vi "convert RegisterMap to FPGA Scalar.vi"(8 "error in":errorcluster, 11 "RegisterMap":T1[](array[typedef]) {"Address" format="%.0x"}) -> (0 "error out":errorcluster, 3 "FPGA Scalar":T6[](array[typedef]) {"Data Type" format="%.0x"})   [LabVIEW 2016, in "FPGA Addon Shared.lvlib"]
uses:
  Shared/FPGA Addon Shared.lvlib
  Shared/Register Information.ctl
  Shared/Data Type.ctl
  <vilib>/rvi/Bitfile/nirviControlStructure.ctl
  <vilib>/rvi/Bitfile/nirviTypdefDescription.ctl
  <vilib>/rvi/Bitfile/nirviMechanicalAction.ctl
  <vilib>/rvi/Bitfile/nirviSubControlStructure.ctl
  <vilib>/rvi/Bitfile/nirviClusterElementControl.ctl
  FPGA/Speciality IO/Types/PWM.Measure.Analog.Measurement.ctl
  FPGA/Speciality IO/Types/PWM.Measure.Digital.Measurement.ctl
  FPGA/Speciality IO/Types/PWM.Generate.Digital.Settings.ctl
  FPGA/Speciality IO/Types/PWM.Measure.Analog.Settings.ctl
  FPGA/Speciality IO/Types/PWM.Measure.Digital.Settings.ctl
  FPGA/Speciality IO/Types/Sine.Generate.Settings.ctl
  FPGA/Speciality IO/Speciality FPGA IO.lvlib
  <vilib>/Utility/Data Type/NI_Data Type.lvlib
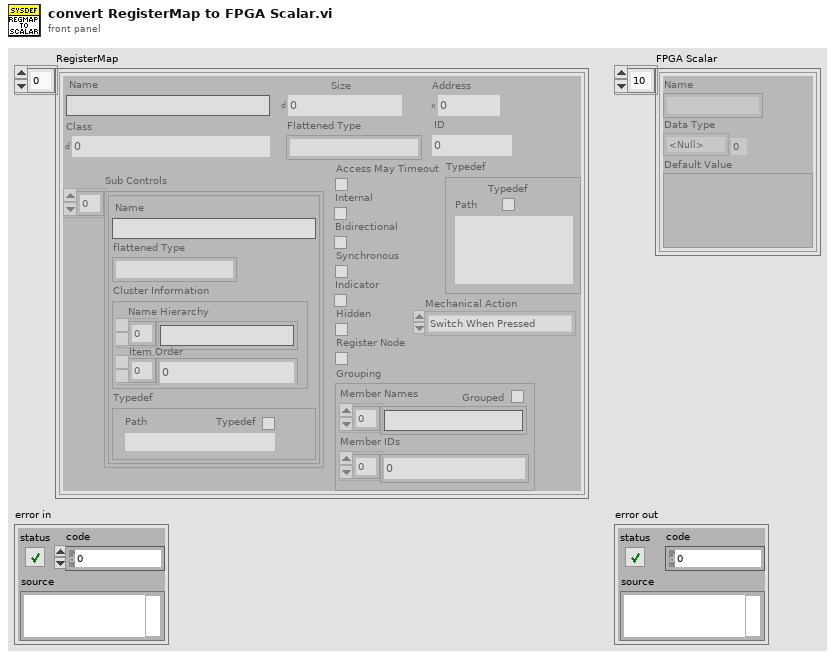
[diagram p1: front panel]
types:
  T1 = typedef "nirviControlStructure.ctl" = cluster{"Name":string, "Hidden":bool, "Indicator":bool, "Flattened Type":string, "Grouping":cluster{"Grouped":bool, "Member Names":string[], "Member IDs":u32[]}, "Address":u32, "Size":u32, "Class":u32, "Internal":bool, "Typedef":T2, "ID":u32, "Bidirectional":bool, "Synchronous":bool, "Mechanical Action":T3, "Sub Controls":T4[], "Access May Timeout":bool, "Register Node":bool}
  T2 = typedef "nirviTypdefDescription.ctl" = cluster{"Typedef":bool, "Path":path}
  T3 = typedef "nirviMechanicalAction.ctl" = enum8{"Switch When Pressed", "Switch When Released", "Switch Until Released", "Latch When Pressed", "Latch When Released", "Latch Until Released"}
  T4 = typedef "nirviSubControlStructure.ctl" = cluster{"Name":string, "flattened Type":string, "Cluster Information":T5, "Typedef":T2}
  T5 = typedef "nirviClusterElementControl.ctl" = cluster{"Name Hierarchy":string[], "Item Order":u32[]}
  T6 = typedef "FPGA Addon Shared.lvlib/Register Information.ctl" = cluster{"Name":string, "Data Type":T7, "Default Value":variant}
  T7 = typedef "FPGA Addon Shared.lvlib/Data Type.ctl" = enum8{"<Null>", "I8", "I16", "I32", "I64", "U8", "U16", "U32", "U64", "SGL", "Boolean", "Analog PWM In Settings", "Analog PWM In", "Digital PWM In Settings", "Digital PWM In", "Digital PWM Out", "Sine Out", "FXP+/-24.5", "FXP+/-16.5", "FXP+/-32.8", "FXP+/-64.32", "FXP+/-16.7", "FXP+/-20.5"}
  T8 = typedef "Speciality FPGA IO.lvlib/PWM.Measure.Digital.Measurement.ctl" = cluster{"ACTIVE TICKS":u32, "INACTIVE TICKS":u32, "ACQ TICKS":u32}
  T9 = typedef "Speciality FPGA IO.lvlib/PWM.Measure.Analog.Measurement.ctl" = cluster{"ACTIVE TICKS":u32, "INACTIVE TICKS":u32, "ACQ TICKS":u32, "ACTIVE VOLTAGE":fxp<+/-,32,8>, "INACTIVE VOLTAGE":fxp<+/-,32,8>}
  T10 = typedef "Speciality FPGA IO.lvlib/Sine.Generate.Settings.ctl" = cluster{"AMP":fxp<+/-,32,8>, "OFFSET":fxp<+/-,32,8>, "PERIODS/TICKS":fxp<+,32,0>}
  T11 = typedef "Speciality FPGA IO.lvlib/PWM.Measure.Digital.Settings.ctl" = cluster{"ACTIVE EDGE":bool, "TIMEOUT":u32}
  T12 = typedef "Speciality FPGA IO.lvlib/PWM.Measure.Analog.Settings.ctl" = cluster{"ACTIVE EDGE":bool, "TIMEOUT":u32, "THRESHOLD":fxp<+/-,32,8>}
  T13 = typedef "Speciality FPGA IO.lvlib/PWM.Generate.Digital.Settings.ctl" = cluster{"ACTIVE EDGE":bool, "ACTIVE TICKS":u32, "INACTIVE TICKS":u32}
  T14 = typedef "NI_Data Type.lvlib/Data Type.ctl" = enum8{"Invalid Type", "Void", "I8", "I16", "I32", "I64", "U8", "U16", "U32", "U64", "Single Float", "Double Float", "Extended Float", "Single Complex", "Double Complex", "Extended Complex", "Enum U8", "Enum U16", "Enum U32", "Enum U64", "Single Float With Unit", "Double Float With Unit", "Extended Float With Unit", "Single Complex with Unit", "Double Complex with Unit", "Extended Complex with Unit", "Boolean", "String", "Path", "Picture", "Tag", "Array", "Cluster", "Variant", "LV Variant", "Waveform", "Timestamp", "Digital Waveform", "Digital Data", "ExpressData", "Refnum", "External Data", "VI", "Poly VI", "LabVIEW Class Instance", "Fixed Point"}
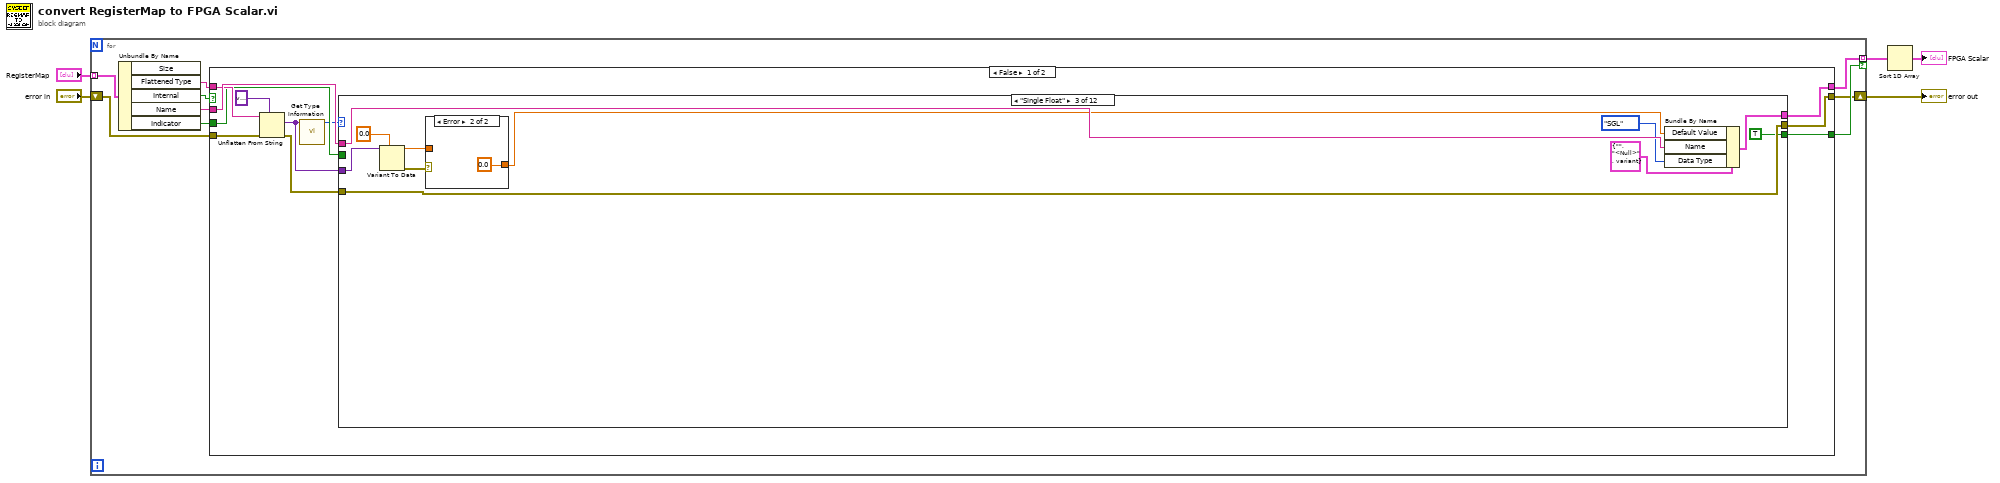
[diagram p0: block diagram]
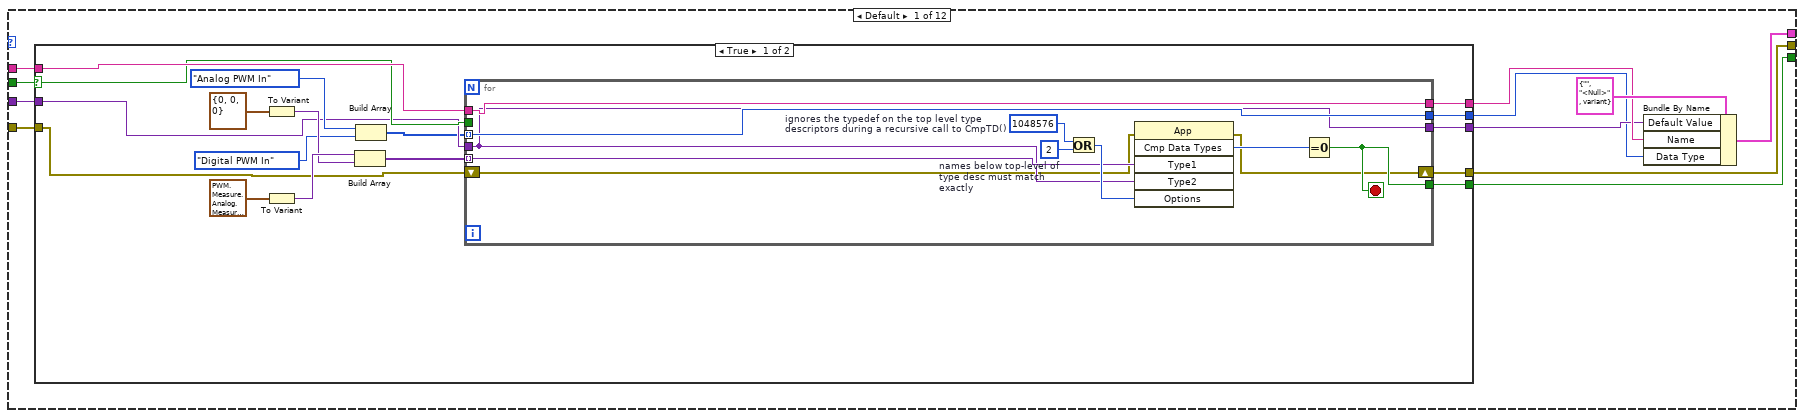
[diagram p2: hidden frame]
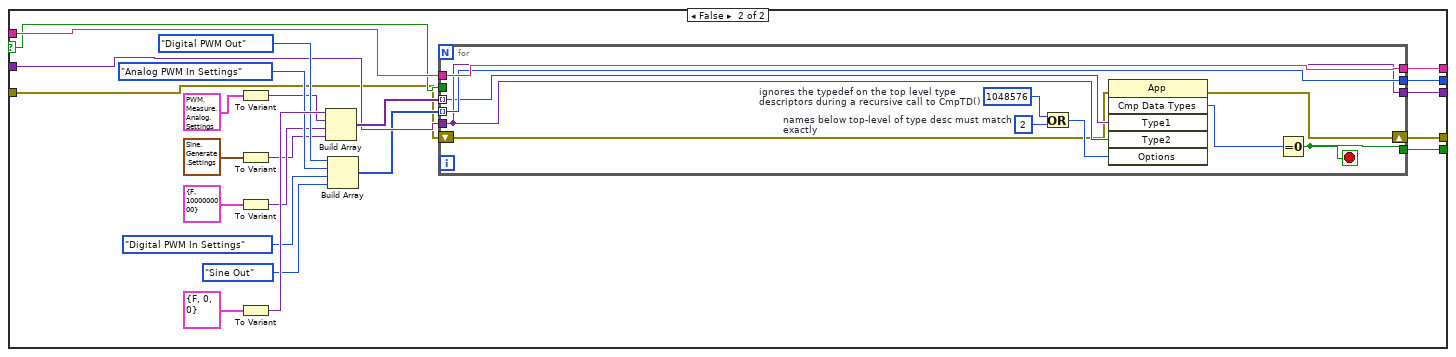
[diagram p3: hidden frame]
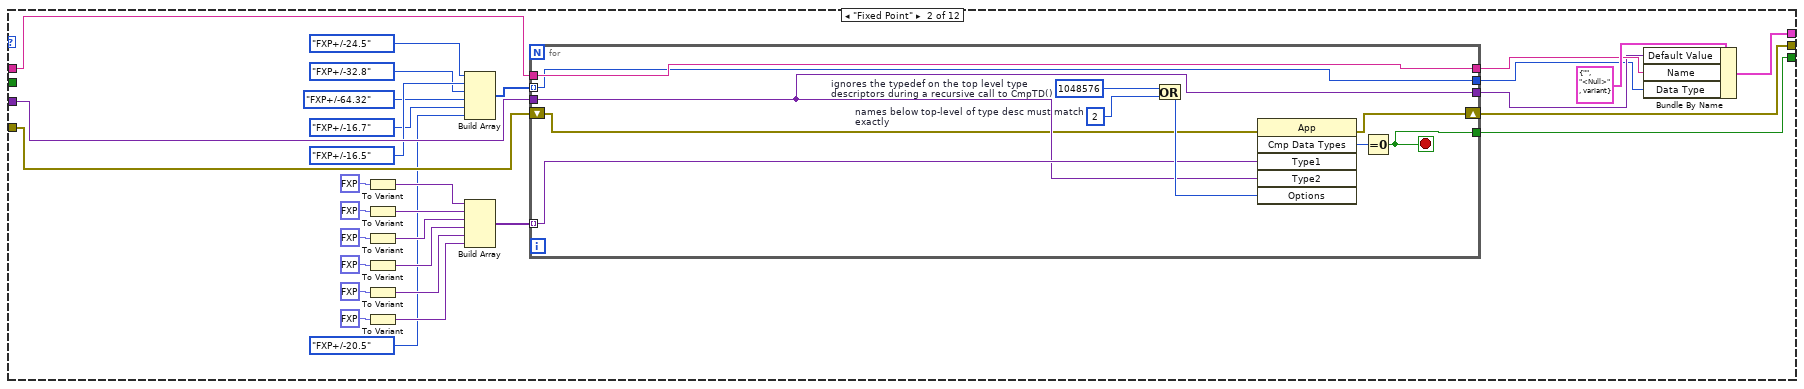
[diagram p4: hidden frame]
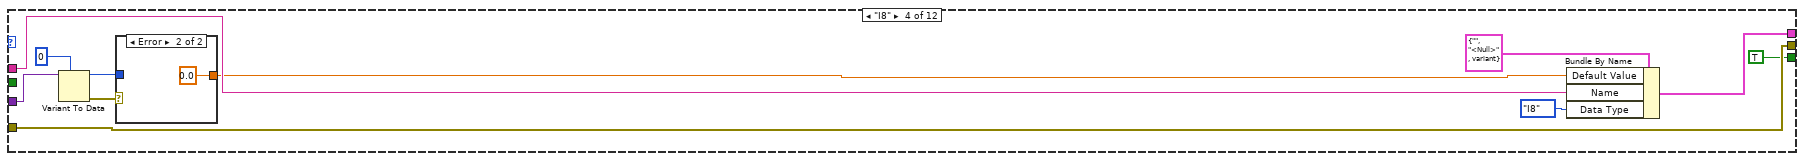
[diagram p6: hidden frame]
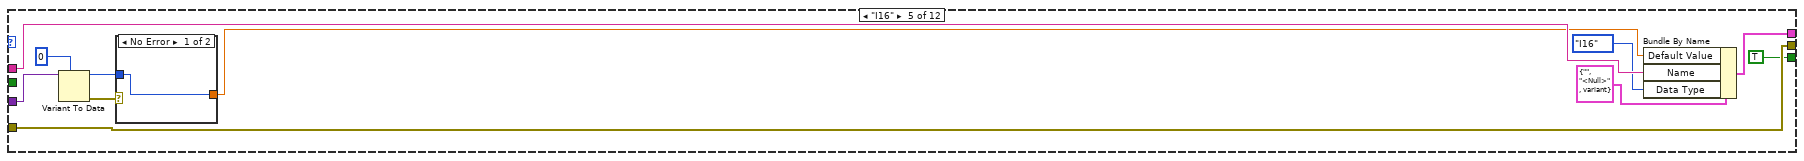
[diagram p8: hidden frame]
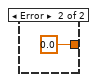
[diagram p9: hidden frame]
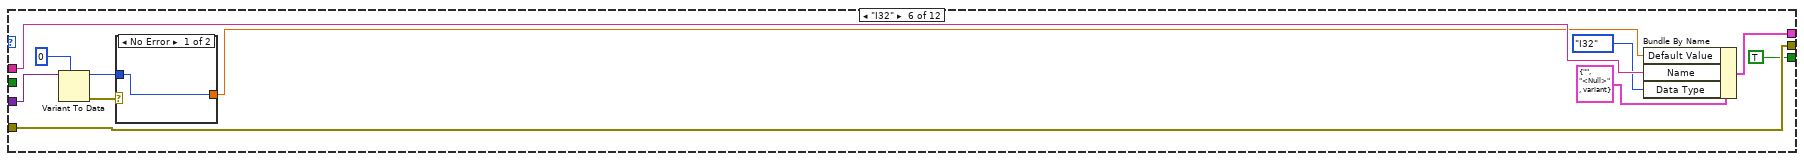
[diagram p10: hidden frame]
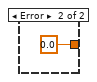
[diagram p11: hidden frame]
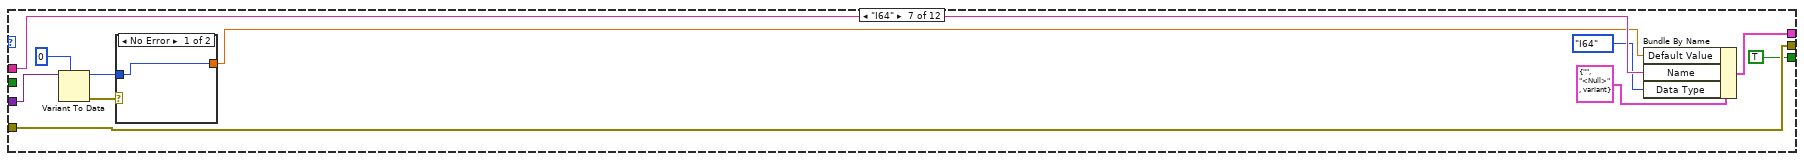
[diagram p12: hidden frame]
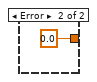
[diagram p13: hidden frame]
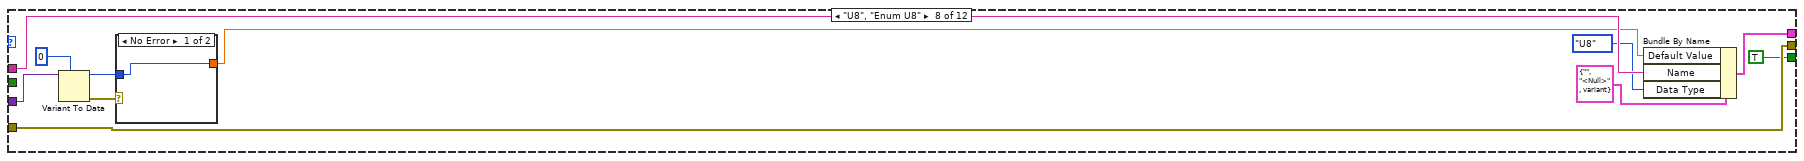
[diagram p14: hidden frame]
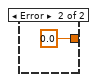
[diagram p15: hidden frame]
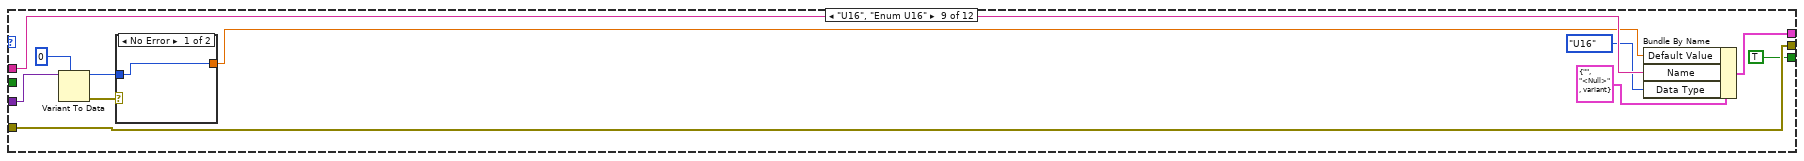
[diagram p16: hidden frame]
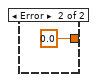
[diagram p17: hidden frame]
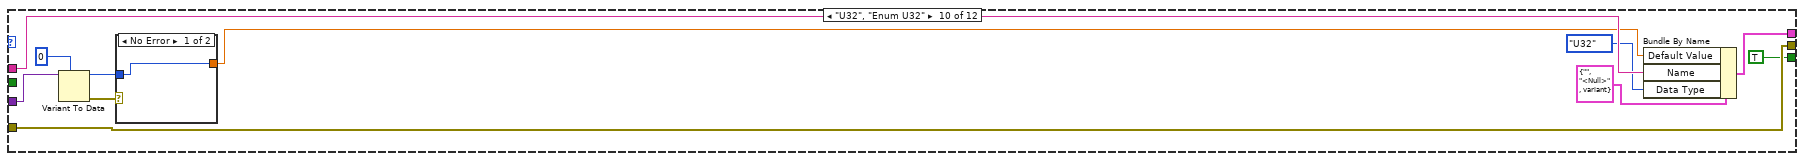
[diagram p18: hidden frame]
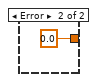
[diagram p19: hidden frame]
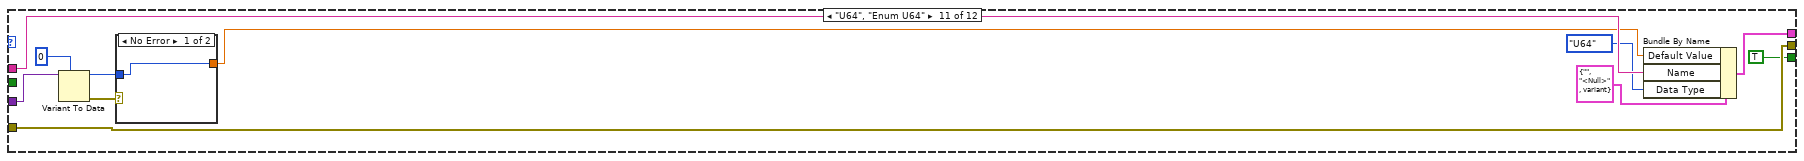
[diagram p20: hidden frame]
diagram:
  n1 = for {
    tunnel: "RegisterMap" -> [w10] mode=indexing
    tunnel: [w14] -> w5 mode=indexing if=w13
    shift-right: [w12] -> w3
    shift-left: "error in" -> [w11]
    n2 = Unbundle By Name(w10) -> ("Flattened Type"=w7:string, "Internal"=w8:bool, "Name"=w9:string, "Indicator"=w6:bool)  [unwired: 1 out]
    n3 = case shown="False" w8 {
      tunnel: w9 -> [w25 _]
      tunnel: [w24 _] -> w14
      tunnel: [w23 FALSE ("Boolean")] -> w13
      tunnel: w7 -> [w20 _]
      tunnel: [w22 w271] -> w12
      tunnel: w11 -> [w19 w271]
      tunnel: w6 -> [w17 _]
      frame False {
        n4 = Unflatten From String(type=variant ("Variant"), binary string=w20, error in (no error)=w19) -> (value=w16:variant, error out=w18:errorcluster)  [unwired: 3 out]
        n5 = call <vilib>:"Get Type Information.vi"("Variant"=w16) -> ("Type"=w15:T14)  [unwired: 6 in, 4 out]
        n6 = case shown="\"Single Float\"" w15 {
          tunnel: [w36 w128 TRUE ("Boolean") TRUE ("Boolean") TRUE ("Boolean") TRUE ("Boolean") TRUE ("Boolean") TRUE ("Boolean") TRUE ("Boolean") TRUE ("Boolean") TRUE ("Boolean") TRUE ("Boolean")] -> w23
          tunnel: w25 -> [w33 w125 w149 w162 w175 w188 w201 w214 w227 w240 w253 w266]
          tunnel: [w34 w126 w148 w161 w174 w187 w200 w213 w226 w239 w252 w265] -> w24
          tunnel: w16 -> [w32 w124 w147 w160 w173 w186 w199 w212 w225 w238 w251 w264]
          tunnel: [w28 w120 w141 w154 w167 w180 w193 w206 w219 w232 w245 w258] -> w22
          tunnel: w18 -> [w27 w119 w141 w154 w167 w180 w193 w206 w219 w232 w245 w258]
          tunnel: w17 -> [w26 _ _ _ _ _ _ _ _ _ _ _]
          frame Default {
            n7 = case shown="True" w26 {
              selector: w26 -> [w49 w84]
              tunnel: [w53 w87] -> w36
              tunnel: w33 -> [w52 w86]
              tunnel: w32 -> [w43 w80]
              tunnel: [w42 w79] -> w31
              tunnel: [w41 w78] -> w30
              tunnel: [w40 w77] -> w29
              tunnel: [w38 w68] -> w28
              tunnel: w27 -> [w37 w69]
              frame True {
                n8 = To Variant(anything=T8 {"ACTIVE TICKS"=0, "INACTIVE TICKS"=0, "ACQ TICKS"=0} ("Cached.Data")) -> (Variant=w47:variant)
                n9 = To Variant(anything=T9 {"ACTIVE TICKS"=0, "INACTIVE TICKS"=0, "ACQ TICKS"=0, "ACTIVE VOLTAGE"=0.0, "INACTIVE VOLTAGE"=0.0} ("Cached.Data")) -> (Variant=w48:variant)
                n10 = Build Array(w48, w47) -> (w44:variant[])
                n11 = Build Array(Data_Type."Analog PWM In" ("Data Type"), Data_Type."Digital PWM In" ("Data Type")) -> (w39:T7[])
                n12 = for {
                  tunnel: w43 -> [w57]
                  tunnel: w52 -> [w64]
                  tunnel: w44 -> [w59] mode=indexing
                  tunnel: [w57] -> w41
                  tunnel: [w64] -> w42
                  tunnel: [w63] -> w40
                  tunnel: w39 -> [w63] mode=indexing
                  tunnel: w49 -> [_]
                  tunnel: [w58] -> w53
                  shift-right: [w54] -> w38
                  shift-left: w37 -> [w55]
                  stop <- w58 stop-if-true
                  w56 = 2  # names below top-level of type desc must match exactly
                  w61 = 1048576  # ignores the typedef on the top level type descriptors during a recursive call to CmpTD()
                  n13 = Or(x=w61, y=w56) -> (x .or. y?=w62:i32)
                  n14 = invoke class="App" method="Cmp Data Types"(error in=w55, "Type1"=w59, "Type2"=w57, "Options"=w62) -> (error out=w54:errorcluster, "Compare Data Types"=w60:i32)  [unwired: 2 in, 4 out]
                  n15 = Equal To 0?(x=w60) -> (x = 0?=w58:bool)
                }
              }
              frame False {
                n16 = To Variant(anything=T12 {"ACTIVE EDGE"=FALSE, "TIMEOUT"=1000000000, "THRESHOLD"=3.0} ("Channel.Settings")) -> (Variant=w73:variant)
                n17 = To Variant(anything=T10 {"AMP"=0.0, "OFFSET"=0.0, "PERIODS/TICKS"=0.0002500000409781933} ("Settings")) -> (Variant=w66:variant)
                n18 = To Variant(anything=T11 {"ACTIVE EDGE"=FALSE, "TIMEOUT"=1000000000} ("Channel.Settings")) -> (Variant=w72:variant)
                n19 = To Variant(anything=T13 {"ACTIVE EDGE"=FALSE, "ACTIVE TICKS"=0, "INACTIVE TICKS"=0} ("Channel.Settings")) -> (Variant=w83:variant)
                n20 = Build Array(w83, w73, w72, w66) -> (w81:variant[])
                n21 = Build Array(Data_Type."Digital PWM Out" ("Data Type"), Data_Type."Analog PWM In Settings" ("Data Type"), Data_Type."Digital PWM In Settings" ("Data Type"), Data_Type."Sine Out" ("Data Type")) -> (w76:T7[])
                n22 = for {
                  tunnel: w80 -> [w93]
                  tunnel: w86 -> [w98]
                  tunnel: w81 -> [w92] mode=indexing
                  tunnel: [w93] -> w78
                  tunnel: [w98] -> w79
                  tunnel: [w97] -> w77
                  tunnel: w76 -> [w97] mode=indexing
                  tunnel: w84 -> [_]
                  tunnel: [w90] -> w87
                  shift-right: [w88] -> w68
                  shift-left: w69 -> [w89]
                  stop <- w90 stop-if-true
                  w95 = 2  # names below top-level of type desc must match exactly
                  w94 = 1048576  # ignores the typedef on the top level type descriptors during a recursive call to CmpTD()
                  n23 = Or(x=w94, y=w95) -> (x .or. y?=w96:i32)
                  n24 = invoke class="App" method="Cmp Data Types"(error in=w89, "Type1"=w92, "Type2"=w93, "Options"=w96) -> (error out=w88:errorcluster, "Compare Data Types"=w91:i32)  [unwired: 2 in, 4 out]
                  n25 = Equal To 0?(x=w91) -> (x = 0?=w90:bool)
                }
              }
            }
            n26 = Bundle By Name(cluster=T6 {"Name"="", "Data Type"=enum."<Null>", "Default Value"=variant(refnum<class> refnum)}, "Default Value"=w30, "Name"=w31, "Data Type"=w29) -> (w34:T6)
          }
          frame "Fixed Point" {
            n27 = To Variant(anything=fxp<+/-,24,5> 0.0 ("Numeric 1 In")) -> (Variant=w118:variant)
            n28 = To Variant(anything=fxp<+/-,16,5> 0.0 ("Numeric 2 In")) -> (Variant=w117:variant)
            n29 = To Variant(anything=fxp<+/-,32,8> 0.0 ("Numeric 3 In")) -> (Variant=w110:variant)
            n30 = To Variant(anything=fxp<+/-,64,32> 0.0 ("Numeric 4 In")) -> (Variant=w109:variant)
            n31 = To Variant(anything=fxp<+/-,16,7> 0.0 ("Numeric 4 In")) -> (Variant=w103:variant)
            n32 = To Variant(anything=fxp<+/-,20,5> 0.0 ("Numeric 4 In")) -> (Variant=w100:variant)
            n33 = Build Array(Data_Type."FXP+/-24.5" ("Data Type"), Data_Type."FXP+/-16.5" ("Data Type"), Data_Type."FXP+/-32.8" ("Data Type"), Data_Type."FXP+/-64.32" ("Data Type"), Data_Type."FXP+/-16.7" ("Data Type"), Data_Type."FXP+/-20.5" ("Data Type")) -> (w113:T7[])
            n34 = Build Array(w118, w117, w110, w109, w103, w100) -> (w114:variant[])
            n35 = for {
              tunnel: w124 -> [w132]
              tunnel: w125 -> [w139]
              tunnel: w114 -> [w134] mode=indexing
              tunnel: [w132] -> w122
              tunnel: [w139] -> w123
              tunnel: [w138] -> w121
              tunnel: w113 -> [w138] mode=indexing
              tunnel: [w133] -> w128
              shift-right: [w129] -> w120
              shift-left: w119 -> [w130]
              stop <- w133 stop-if-true
              w131 = 2  # names below top-level of type desc must match exactly
              w136 = 1048576  # ignores the typedef on the top level type descriptors during a recursive call to CmpTD()
              n36 = Or(x=w136, y=w131) -> (x .or. y?=w137:i32)
              n37 = invoke class="App" method="Cmp Data Types"(error in=w130, "Type1"=w134, "Type2"=w132, "Options"=w137) -> (error out=w129:errorcluster, "Compare Data Types"=w135:i32)  [unwired: 2 in, 4 out]
              n38 = Equal To 0?(x=w135) -> (x = 0?=w133:bool)
            }
            n39 = Bundle By Name(cluster=T6 {"Name"="", "Data Type"=enum."<Null>", "Default Value"=variant(refnum<class> refnum)}, "Default Value"=w122, "Name"=w123, "Data Type"=w121) -> (w126:T6)
          }
          frame "Single Float" {
            n40 = Variant To Data(type=sgl 0.0, Variant=w147) -> (data=w143:sgl, error out=w145:errorcluster)  [unwired: 1 in]
            n41 = case shown="Error" w145 {
              tunnel: [w151 0.0] -> w144
              tunnel: w143 -> [w151 _]
              frame No Error {
              }
              frame Error {
              }
            }
            n42 = Bundle By Name(cluster=T6 {"Name"="", "Data Type"=enum."<Null>", "Default Value"=variant(refnum<class> refnum)}, "Default Value"=w144, "Name"=w149, "Data Type"=Data_Type."SGL") -> (w148:T6)
          }
          frame "I8" {
            n43 = Variant To Data(type=i8 0, Variant=w160) -> (data=w156:i8, error out=w158:errorcluster)  [unwired: 1 in]
            n44 = case shown="Error" w158 {
              tunnel: [w164 0.0] -> w157
              tunnel: w156 -> [w164 _]
              frame No Error {
              }
              frame Error {
              }
            }
            n45 = Bundle By Name(cluster=T6 {"Name"="", "Data Type"=enum."<Null>", "Default Value"=variant(refnum<class> refnum)}, "Default Value"=w157, "Name"=w162, "Data Type"=Data_Type."I8") -> (w161:T6)
          }
          frame "I16" {
            n46 = Variant To Data(type=i16 0, Variant=w173) -> (data=w169:i16, error out=w171:errorcluster)  [unwired: 1 in]
            n47 = case shown="No Error" w171 {
              tunnel: [w177 0.0] -> w170
              tunnel: w169 -> [w177 _]
              frame No Error {
              }
              frame Error {
              }
            }
            n48 = Bundle By Name(cluster=T6 {"Name"="", "Data Type"=enum."<Null>", "Default Value"=variant(refnum<class> refnum)}, "Default Value"=w170, "Name"=w175, "Data Type"=Data_Type."I16") -> (w174:T6)
          }
          frame "I32" {
            n49 = Variant To Data(type=0, Variant=w186) -> (data=w182:i32, error out=w184:errorcluster)  [unwired: 1 in]
            n50 = case shown="No Error" w184 {
              tunnel: [w190 0.0] -> w183
              tunnel: w182 -> [w190 _]
              frame No Error {
              }
              frame Error {
              }
            }
            n51 = Bundle By Name(cluster=T6 {"Name"="", "Data Type"=enum."<Null>", "Default Value"=variant(refnum<class> refnum)}, "Default Value"=w183, "Name"=w188, "Data Type"=Data_Type."I32") -> (w187:T6)
          }
          frame "I64" {
            n52 = Variant To Data(type=i64 0, Variant=w199) -> (data=w195:i64, error out=w197:errorcluster)  [unwired: 1 in]
            n53 = case shown="No Error" w197 {
              tunnel: [w203 0.0] -> w196
              tunnel: w195 -> [w203 _]
              frame No Error {
              }
              frame Error {
              }
            }
            n54 = Bundle By Name(cluster=T6 {"Name"="", "Data Type"=enum."<Null>", "Default Value"=variant(refnum<class> refnum)}, "Default Value"=w196, "Name"=w201, "Data Type"=Data_Type."I64") -> (w200:T6)
          }
          frame "U8", "Enum U8" {
            n55 = Variant To Data(type=u8 0, Variant=w212) -> (data=w208:u8, error out=w210:errorcluster)  [unwired: 1 in]
            n56 = case shown="No Error" w210 {
              tunnel: [w216 0.0] -> w209
              tunnel: w208 -> [w216 _]
              frame No Error {
              }
              frame Error {
              }
            }
            n57 = Bundle By Name(cluster=T6 {"Name"="", "Data Type"=enum."<Null>", "Default Value"=variant(refnum<class> refnum)}, "Default Value"=w209, "Name"=w214, "Data Type"=Data_Type."U8") -> (w213:T6)
          }
          frame "U16", "Enum U16" {
            n58 = Variant To Data(type=u16 0, Variant=w225) -> (data=w221:u16, error out=w223:errorcluster)  [unwired: 1 in]
            n59 = case shown="No Error" w223 {
              tunnel: [w229 0.0] -> w222
              tunnel: w221 -> [w229 _]
              frame No Error {
              }
              frame Error {
              }
            }
            n60 = Bundle By Name(cluster=T6 {"Name"="", "Data Type"=enum."<Null>", "Default Value"=variant(refnum<class> refnum)}, "Default Value"=w222, "Name"=w227, "Data Type"=Data_Type."U16") -> (w226:T6)
          }
          frame "U32", "Enum U32" {
            n61 = Variant To Data(type=u32 0, Variant=w238) -> (data=w234:u32, error out=w236:errorcluster)  [unwired: 1 in]
            n62 = case shown="No Error" w236 {
              tunnel: [w242 0.0] -> w235
              tunnel: w234 -> [w242 _]
              frame No Error {
              }
              frame Error {
              }
            }
            n63 = Bundle By Name(cluster=T6 {"Name"="", "Data Type"=enum."<Null>", "Default Value"=variant(refnum<class> refnum)}, "Default Value"=w235, "Name"=w240, "Data Type"=Data_Type."U32") -> (w239:T6)
          }
          frame "U64", "Enum U64" {
            n64 = Variant To Data(type=u64 0, Variant=w251) -> (data=w247:u64, error out=w249:errorcluster)  [unwired: 1 in]
            n65 = case shown="No Error" w249 {
              tunnel: [w255 0.0] -> w248
              tunnel: w247 -> [w255 _]
              frame No Error {
              }
              frame Error {
              }
            }
            n66 = Bundle By Name(cluster=T6 {"Name"="", "Data Type"=enum."<Null>", "Default Value"=variant(refnum<class> refnum)}, "Default Value"=w248, "Name"=w253, "Data Type"=Data_Type."U64") -> (w252:T6)
          }
          frame "Boolean" {
            n67 = Variant To Data(type=FALSE, Variant=w264) -> (data=w260:bool, error out=w262:errorcluster)  [unwired: 1 in]
            n68 = case shown="No Error" w262 {
              tunnel: [w268 0.0] -> w261
              tunnel: w260 -> [w269 _]
              frame No Error {
                n69 = Boolean To (0,1)(Boolean=w269) -> (0, 1=w268:i16)
              }
              frame Error {
              }
            }
            n70 = Bundle By Name(cluster=T6 {"Name"="", "Data Type"=enum."<Null>", "Default Value"=variant(refnum<class> refnum)}, "Default Value"=w261, "Name"=w266, "Data Type"=Data_Type."Boolean") -> (w265:T6)
          }
        }
      }
      frame True {
      }
    }
  }
  "error out" <- w3
  n71 = Sort 1D Array(array=w5) -> (sorted array=→"FPGA Scalar":T6[])
